vi "二维数组行交换并重新赋初值 (子VI).vi"(11 "输出数组 3":string[][](array[string])) -> (3 "输出数组 2":string[][](array[string]))   [LabVIEW 2016]
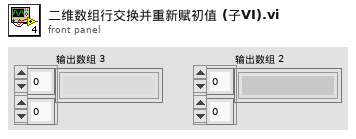
[diagram p1: front panel]
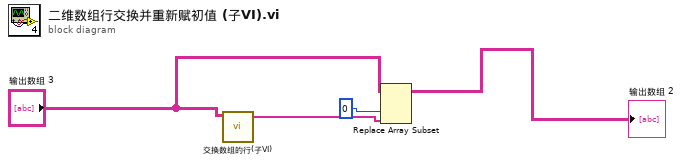
[diagram p0: block diagram]
diagram:
  n1 = call "交换数组的行(子VI).vi"("输出数组输入"="输出数组 3") -> ("数组"=w2:string[])  [unwired: 10 in]
  n2 = Replace Array Subset(array="输出数组 3", new element=w2, index (col)=0 ("禁用的索引 (列)")) -> (→"输出数组 2":string[][])  [unwired: 1 in]
